vi "Cp&Cpk.vi"(6 "Sigma tolerance (6)":dbl=6.0, 7 "Sigma":dbl, 8 "Error In":errorcluster, 9 "Low limit":dbl, 10 "High limit":dbl, 11 "Mean":dbl) -> (0 "Error Out":errorcluster, 1 "PPM":dbl, 2 "Ppk/Cpk/Cmk":dbl, 3 "Pp/Cp/Cm":dbl)   [LabVIEW 2019, in "Tools.lvlib"]
uses:
  <vilib>/gmath/statdist.llb/Normal CDF.vi
  Tools.lvlib
  <vilib>/gmath/NI_Gmath.lvlib
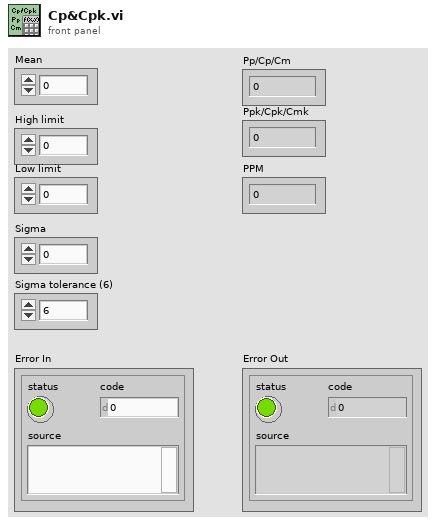
[diagram p1: front panel]
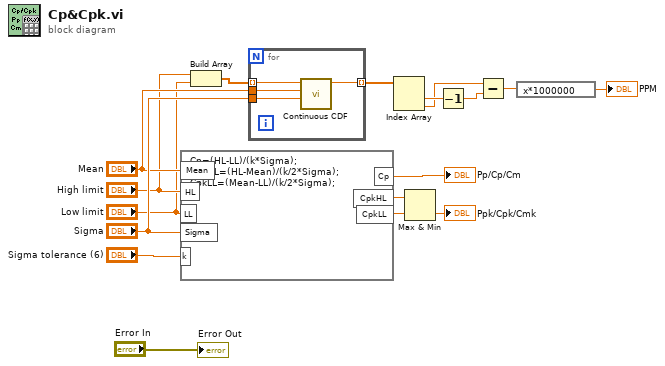
[diagram p0: block diagram]
diagram:
  n1 = formula code="Cp=(HL-LL)/(k*Sigma);\nCpkHL=(HL-Mean)/(k/2*Sigma);\nCpkLL=(Mean-LL)/(k/2*Sigma);"("Mean"="Mean", "LL"="Low limit", "HL"="High limit", "Sigma"="Sigma", "k"="Sigma tolerance (6)") -> ("Cp"=→"Pp/Cp/Cm":dbl, "CpkHL"=w17:dbl, "CpkLL"=w16:dbl)
  n2 = Build Array("High limit", "Low limit") -> (w7:dbl[])
  n3 = for {
    tunnel: "Sigma" -> [w21]
    tunnel: "Mean" -> [w20]
    tunnel: w7 -> [w19] mode=indexing
    tunnel: [w18] -> w6 mode=indexing
    n4 = call-poly <vilib>:"Continuous CDF.vi"("std"=w21, "mean"=w20, "x"=w19) -> ("cdf(x)"=w18:dbl)  [unwired: 7 in, 1 out]
  }
  n5 = Index Array(array=w6) -> (element #1=w5:dbl, element #2=w4:dbl)  [unwired: 2 in]
  n6 = Max & Min(x=w17, y=w16) -> (min(x,y)=→"Ppk/Cpk/Cmk":dbl)  [unwired: 1 out]
  n7 = Decrement(x=w5) -> (x-1=w3:dbl)
  n8 = Subtract(x=w4, y=w3) -> (x-y=w2:dbl)
  n9 = expression code="x*1000000"(w2) -> (→"PPM":dbl)
  "Error Out" <- "Error In"
